vi "Get Font Settings for VI.vi"(4 "error in (no error)":errorcluster, 7 "Name":string) -> (0 "error out":errorcluster, 2 "Control Names":string[](array[string]), 3 "Font Parameters":cluster{T1[]}[](array[cluster]))   [LabVIEW 2015, in "Config Data.lvlib" / "Config Data.lvclass"]
uses:
  Config Data.lvclass
  Display Properties Manager/_typedefs/Font Parameters.ctl
  Display Properties Manager/_typedefs/Control Component to Set.ctl
  Display Properties Manager/Display Properties Manager.lvlib
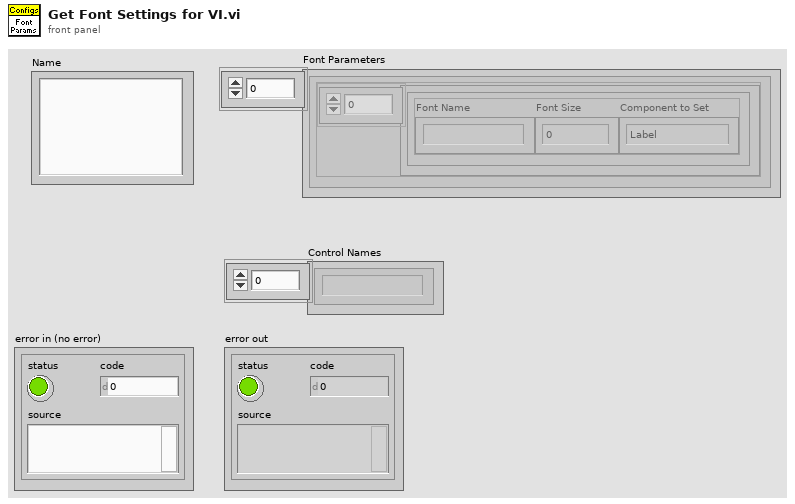
[diagram p1: front panel]
types:
  T1 = typedef "Display Properties Manager.lvlib/Font Parameters.ctl" = cluster{"Font Name":string, "Font Size":u32, "Component to Set":T2}
  T2 = typedef "Display Properties Manager.lvlib/Control Component to Set.ctl" = enum16{"Label", "Caption", "Contents"}
  T3 = cluster{"Font Parameters":cluster{T1[]}[], "Control Names":string[]}
  T4 = cluster{"Font Parameters":cluster{T1[]}[], "Control Names":string[]}[]
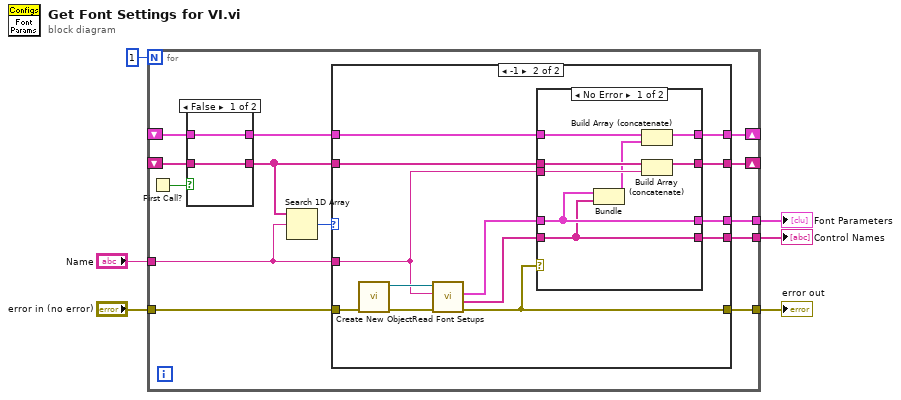
[diagram p0: block diagram]
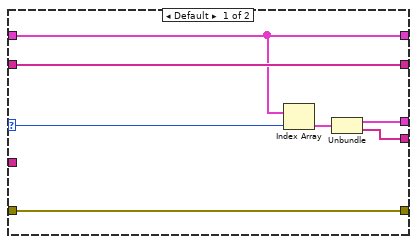
[diagram p3: hidden frame]
diagram:
  n1 = for {
    N: 1 -> [_]
    tunnel: "Name" -> [w12]
    tunnel: [w18] -> w4
    tunnel: [w17] -> w3
    tunnel: "error in (no error)" -> [w19]
    tunnel: [w16] -> w2
    shift-right: [w15] -> _
    shift-left: _ -> [w10]
    shift-right: [w14] -> _
    shift-left: _ -> [w9]
    n2 = First Call?() -> (First Call?: T/F=w11:bool)
    n3 = case shown="False" w11 {
      tunnel: w10 -> [w21 _]
      tunnel: w9 -> [w20 _]
      tunnel: [w20 _] -> w8
      tunnel: [w21 _] -> w7
      frame False {
      }
      frame True {
      }
    }
    n4 = Search 1D Array(1D array=w8, element=w12) -> (index of element=w13:i32)  [unwired: 1 in]
    n5 = case shown="-1" w13 {
      selector: w13 -> [w26 _]
      tunnel: w12 -> [_ w31]
      tunnel: w19 -> [w27 w30]
      tunnel: [w22 w37] -> w18
      tunnel: [w23 w36] -> w17
      tunnel: [w27 w33] -> w16
      tunnel: w8 -> [w28 w41]
      tunnel: w7 -> [w25 w39]
      tunnel: [w25 w38] -> w15
      tunnel: [w28 w40] -> w14
      frame Default {
        n6 = Index Array(array=w25, index=w26) -> (element=w24:T3)
        n7 = Unbundle(w24) -> ("Font Parameters"=w22:cluster{T1[]}[], "Control Names"=w23:string[])
      }
      frame -1 {
        n8 = call "Create New Object.vi"("Error In"=w30) -> ("Error Out"=w29:errorcluster, "Config Data"=w32:refnum<class "Config Data.lvclass">)  [unwired: 5 in]
        n9 = call-dynamic "Read Font Setups.vi"("error in (no error)"=w29, "Owner Name"=w31, "Config Data in"=w32) -> ("error out"=w33:errorcluster, "Control Names"=w34:string[], "Font Parameters"=w35:cluster{T1[]}[])  [unwired: 1 in, 1 out]
        n10 = case shown="No Error" w33 {
          tunnel: w41 -> [w49 w51]
          tunnel: [w48 w51] -> w40
          tunnel: w31 -> [w47 _]
          tunnel: w39 -> [w46 w50]
          tunnel: [w45 w50] -> w38
          tunnel: w35 -> [w43 _]
          tunnel: w34 -> [w42 _]
          tunnel: [w43 _] -> w37
          tunnel: [w42 _] -> w36
          frame No Error {
            n11 = Bundle("Font Parameters"=w43, "Control Names"=w42) -> (w44:T3)  [unwired: 1 in]
            n12 = Build Array (concatenate)(w46, w44) -> (w45:T4)
            n13 = Build Array (concatenate)(w49, w47) -> (w48:string[])
          }
          frame Error {
          }
        }
      }
    }
  }
  "Font Parameters" <- w4
  "Control Names" <- w3
  "error out" <- w2
